vi "last_packet_functional.vi"(7 "MAC Address":string, 10 "Packets":string[](array[string]), 11 "AOL_Globals":T1={"Imaging Protocol"=enum."AOL Z-Stack", "Number of POI"=0, "Number of Miniscans"=0, "Number of Trials"=0, "Number of Cycles "=0, "# Averaged Frames"=0, "Laser power (%)"=0, "Pockels (V)"=0.0, "Acquisition Length (sec)"=0.0, "Fill time (us)"=0.0, "POI Dwell time (us)"=0.0, "Miniscan Dwell time per pixel (us)"=0.0, "PMT 1"=0.0, "PMT 2"=0.0, "Back Apperture (mA)"=0.0, "Frame Size"=0, "Center Frequency"=0.0, "Field of View (norm)"=0.0, "DwellTime (us)"=0.0, "Wavelength (nm)"=0.0, "Zoom"=0.0, "AOL Z"=0.0, "AOL Mode"=enum."Raster", "GridXY"=0.0, "GridZ"=0.0, "TriggerPeriod (sec)"=0.0, "Number of Pixels in Miniscan"=0, "Experiment folder path"=path "", "X centre"=0.0, "Y centre"=0.0, "Angle (degrees)"=0.0, "Plane Mode"=0, "Threshold"=[], "Regenerate Chirps"=FALSE, "Rectangle ROI length (pixels)"=0, "Rectangle ROI height (pixels)"=0, "AOD fill"=4900, "StartupDelay"=0, "Samples Wait after Trigger"=5080, "Slip Cycle"=600000, "Add Cycle"=TRUE, "Functional Mode"=enum."Point", "Z Start"=0.0, "Z Stop"=0.0, "# Planes"=0} {"Plane Mode" items=["XY Plane", "XZ Plane", "YZ Plane", "arbitraryplane"]; "Frame Size" items=["100X100"=100, "128X128"=128, "200X200"=200, "256X256"=256, "512X512"=512, "1024x1024"=1024, "2048x2048"=2048]; "Back Apperture (mA)" format="%#.6g"; "Pockels (V)" format="%#.6g"; "PMT 2" format="%#.6g"; "PMT 1" format="%#.6g"; "Angle (degrees)" format="%#.6g"; "POI Dwell time (us)" format="%#.6g"}) -> (0 "Repeat":i32, 2 "HexPackets":string[](array[string]), 3 "Total Packets":i32)   [LabVIEW 2017]
uses:
  Typedefs/Controls/AOL_Globals.ctl
  Typedefs/Imaging Protocols enum.ctl
  Typedefs/Frame Size.ctl
  Typedefs/AOL modes.ctl
  Typedefs/Plane Mode.ctl
  Typedefs/Functional Mode.ctl
panel:
  # "RE-ENTRANT"
  # "SUB-ROUTINE"
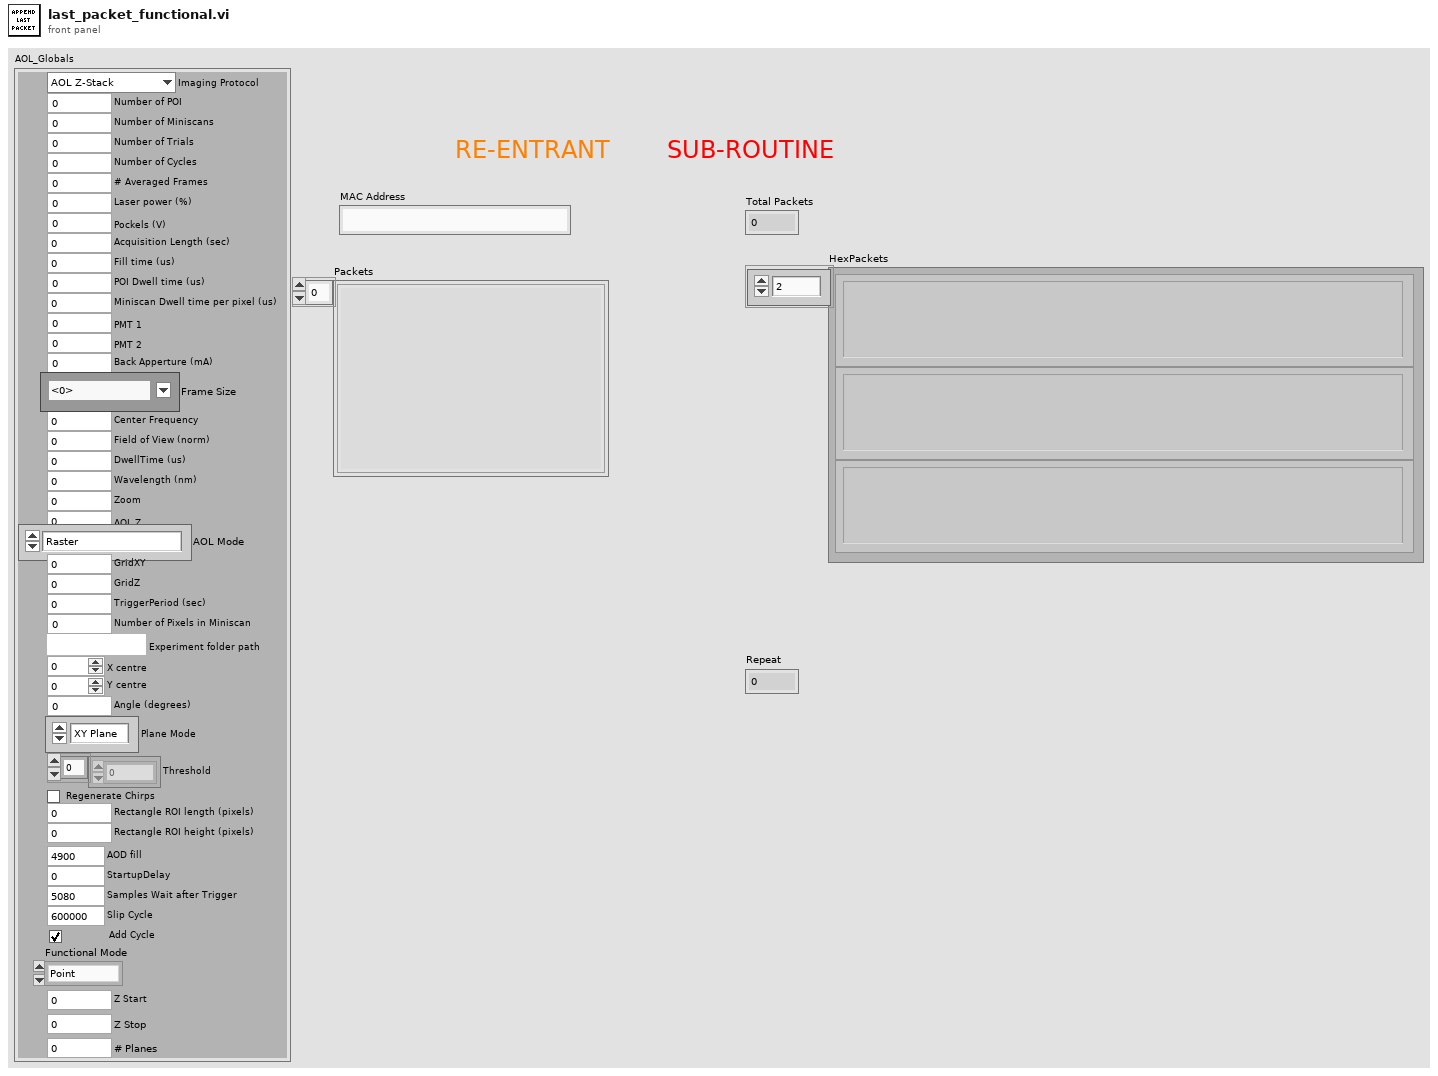
[diagram p1: front panel]
types:
  T1 = typedef "AOL_Globals.ctl" = cluster{"Imaging Protocol":T2, "Number of POI":u16, "Number of Miniscans":u16, "Number of Trials":u16, "Number of Cycles ":u64, "# Averaged Frames":u16, "Laser power (%)":u8, "Pockels (V)":dbl, "Acquisition Length (sec)":dbl, "Fill time (us)":dbl, "POI Dwell time (us)":dbl, "Miniscan Dwell time per pixel (us)":dbl, "PMT 1":dbl, "PMT 2":dbl, "Back Apperture (mA)":dbl, "Frame Size":T3, "Center Frequency":dbl, "Field of View (norm)":dbl, "DwellTime (us)":dbl, "Wavelength (nm)":dbl, "Zoom":dbl, "AOL Z":dbl, "AOL Mode":T4, "GridXY":dbl, "GridZ":dbl, "TriggerPeriod (sec)":dbl, "Number of Pixels in Miniscan":u16, "Experiment folder path":path, "X centre":dbl, "Y centre":dbl, "Angle (degrees)":dbl, "Plane Mode":T5, "Threshold":u16[], "Regenerate Chirps":bool, "Rectangle ROI length (pixels)":u16, "Rectangle ROI height (pixels)":u16, "AOD fill":u16, "StartupDelay":i32, "Samples Wait after Trigger":u16, "Slip Cycle":u32, "Add Cycle":bool, "Functional Mode":T6, "Z Start":dbl, "Z Stop":dbl, "# Planes":i32}
  T2 = typedef "Imaging Protocols enum.ctl" = enum16{"AOL Z-Stack", "Motor Z Stack", "Functional Acquisition", "Single Plane Acquisition", "Volume Acquisition", "Live Imaging", "Live Plane Imaging", "Live Volume Imaging"}
  T3 = typedef "Frame Size.ctl" = u16
  T4 = typedef "AOL modes.ctl" = enum16{"Raster", "Structural", "Pointing", "Mini Scan", "Alignment"}
  T5 = typedef "Plane Mode.ctl" = u16
  T6 = typedef "Functional Mode.ctl" = enum16{"Point", "Line", "Patch", "Plane", "Volume"}
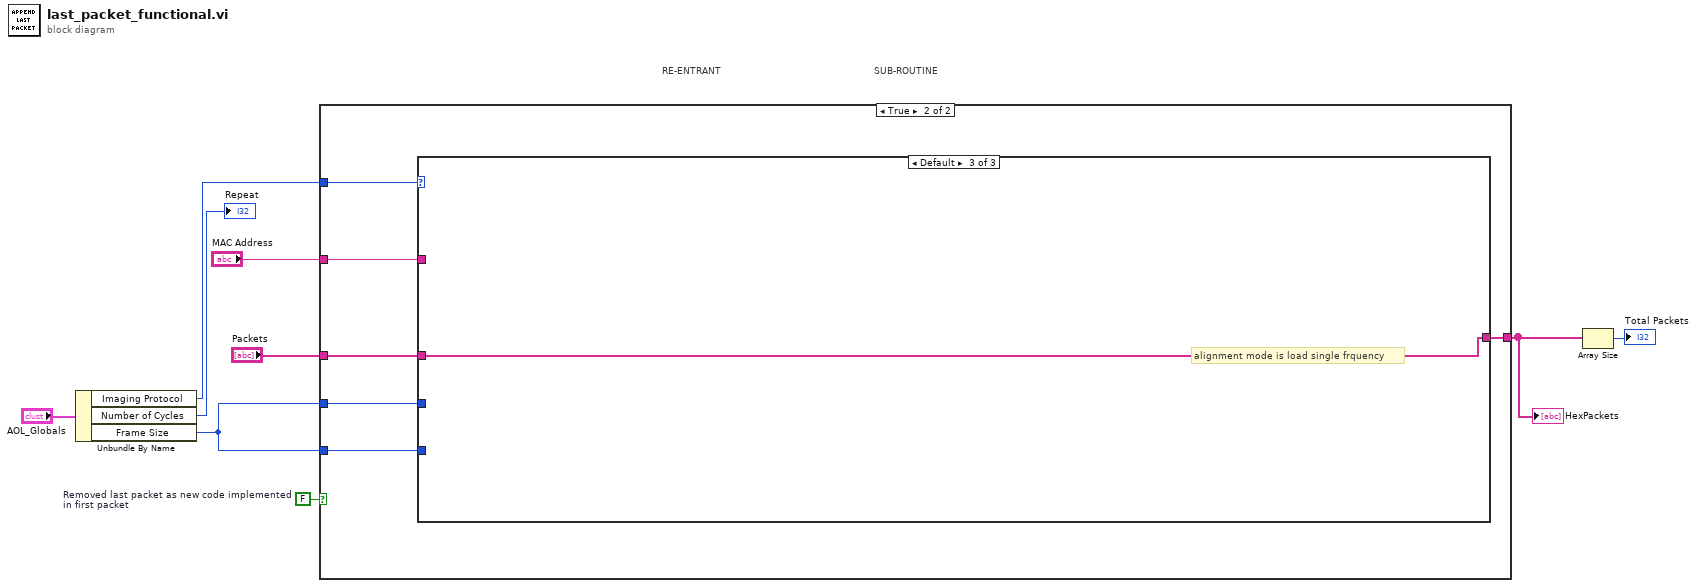
[diagram p0: block diagram]
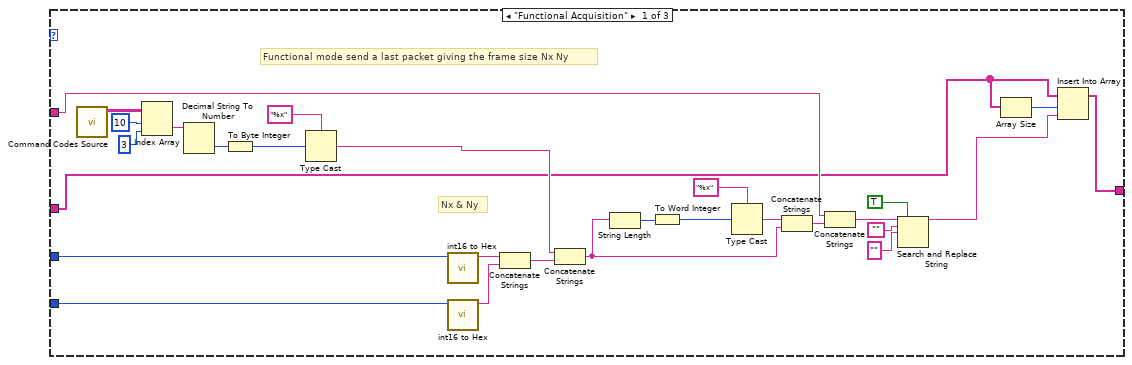
[diagram p3: hidden frame]
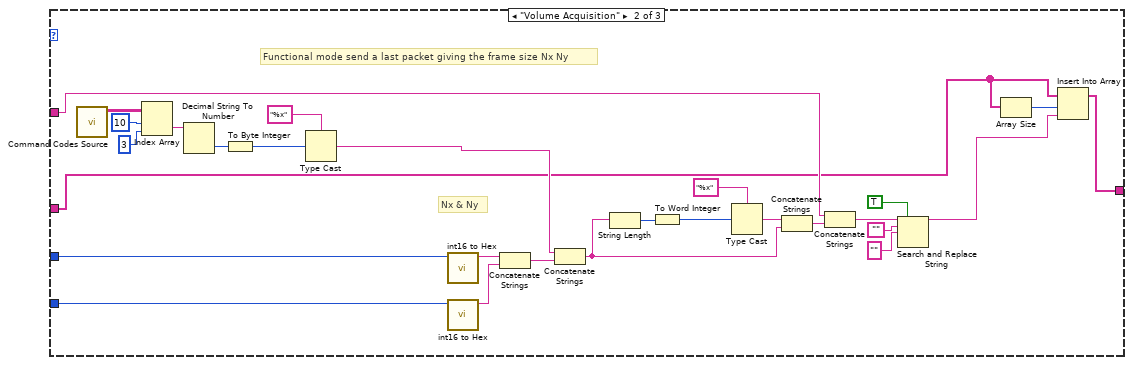
[diagram p4: hidden frame]
diagram:
  w1 = FALSE  # Removed last packet as new code implemented in first packet
  # "SUB-ROUTINE"
  # "RE-ENTRANT"
  n1 = Unbundle By Name("AOL_Globals") -> ("Imaging Protocol"=w4:T2, "Number of Cycles"=→"Repeat":u64, "Frame Size"=w2:T3)
  n2 = case shown="True" w1 {
    tunnel: [w10 w16] -> w8
    tunnel: "MAC Address" -> [_ w15]
    tunnel: "Packets" -> [w10 w14]
    tunnel: w4 -> [_ w13]
    tunnel: w2 -> [_ w12]
    tunnel: w2 -> [_ w11]
    frame False {
    }
    frame True {
      n3 = case shown="Default" w13 {
        tunnel: [w17 w45 w73] -> w16
        tunnel: w11 -> [w24 w52 _]
        tunnel: w12 -> [w23 w51 _]
        tunnel: w14 -> [w18 w46 w73]
        tunnel: w15 -> [w22 w50 _]
        frame "Functional Acquisition" {
          # "Nx & Ny"
          # "Functional mode send a last packet giving the frame size Nx Ny"
          n4 = call "Command Codes Source.vi"() -> ("Commands for FPGA"=w35:string[][])  [unwired: 11 in]
          n5 = Index Array(array=w35, index (row)=10 ("disabled index (row)"), index (col)=3 ("disabled index (col)")) -> (element=w29:string)
          n6 = Decimal String To Number(string=w29) -> (number=w31:i32)  [unwired: 2 in, 1 out]
          n7 = To Byte Integer(number=w31) -> (8bit integer=w30:i8)
          n8 = Type Cast(type="%x", x=w30) -> (*(type *) &x=w21:string)
          n9 = call "int16 to Hex.vi"("number"=w23) -> ("Hex string"=w28:string)  [unwired: 10 in]
          n10 = call "int16 to Hex.vi"("number"=w24) -> ("Hex string"=w27:string)  [unwired: 10 in]
          n11 = Concatenate Strings(w28, w27) -> (w26:string)
          n12 = Concatenate Strings(w21, w26) -> (w25:string)
          n13 = String Length(string=w25) -> (length=w41:i32)
          n14 = To Word Integer(number=w41) -> (16bit integer=w36:i16)
          n15 = Type Cast(type="%x", x=w36) -> (*(type *) &x=w43:string)
          n16 = Concatenate Strings(w43, w25) -> (w44:string)
          n17 = Concatenate Strings(w22, w44) -> (w40:string)
          n18 = Search and Replace String(replace all?=TRUE ("replace all? (F)"), input string=w40, search string="", replace string="" ("replace string (\"\")")) -> (result string=w19:string)  [unwired: 4 in, 3 out]
          n19 = Array Size(array=w18) -> (size(s)=w20:i32)
          n20 = Insert Into Array(array=w18, index=w20, new element=w19) -> (w17:string[])
        }
        frame "Volume Acquisition" {
          # "Nx & Ny"
          # "Functional mode send a last packet giving the frame size Nx Ny"
          n21 = call "Command Codes Source.vi"() -> ("Commands for FPGA"=w63:string[][])  [unwired: 11 in]
          n22 = Index Array(array=w63, index (row)=10 ("disabled index (row)"), index (col)=3 ("disabled index (col)")) -> (element=w57:string)
          n23 = Decimal String To Number(string=w57) -> (number=w59:i32)  [unwired: 2 in, 1 out]
          n24 = To Byte Integer(number=w59) -> (8bit integer=w58:i8)
          n25 = Type Cast(type="%x", x=w58) -> (*(type *) &x=w49:string)
          n26 = call "int16 to Hex.vi"("number"=w51) -> ("Hex string"=w56:string)  [unwired: 10 in]
          n27 = call "int16 to Hex.vi"("number"=w52) -> ("Hex string"=w55:string)  [unwired: 10 in]
          n28 = Concatenate Strings(w56, w55) -> (w54:string)
          n29 = Concatenate Strings(w49, w54) -> (w53:string)
          n30 = String Length(string=w53) -> (length=w69:i32)
          n31 = To Word Integer(number=w69) -> (16bit integer=w64:i16)
          n32 = Type Cast(type="%x", x=w64) -> (*(type *) &x=w71:string)
          n33 = Concatenate Strings(w71, w53) -> (w72:string)
          n34 = Concatenate Strings(w50, w72) -> (w68:string)
          n35 = Search and Replace String(replace all?=TRUE ("replace all? (F)"), input string=w68, search string="", replace string="" ("replace string (\"\")")) -> (result string=w47:string)  [unwired: 4 in, 3 out]
          n36 = Array Size(array=w46) -> (size(s)=w48:i32)
          n37 = Insert Into Array(array=w46, index=w48, new element=w47) -> (w45:string[])
        }
        frame Default {
          # "alignment mode is load single frquency"
        }
      }
    }
  }
  "HexPackets" <- w8
  n38 = Array Size(array=w8) -> (size(s)=→"Total Packets":i32)
